vi "expressions.vi"() -> ()   [LabVIEW 2017]
uses:
  <vilib>/express/express arith-compare/Formula/XNode/ExpressFormulaBlockNode.xnode
panel:
  out "X1 2":dbl
  out "Result":dbl
  out "X1+2":dbl
  in  "X1":dbl
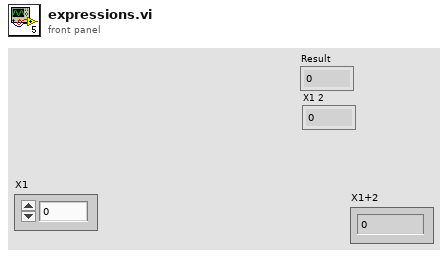
[diagram p1: front panel]
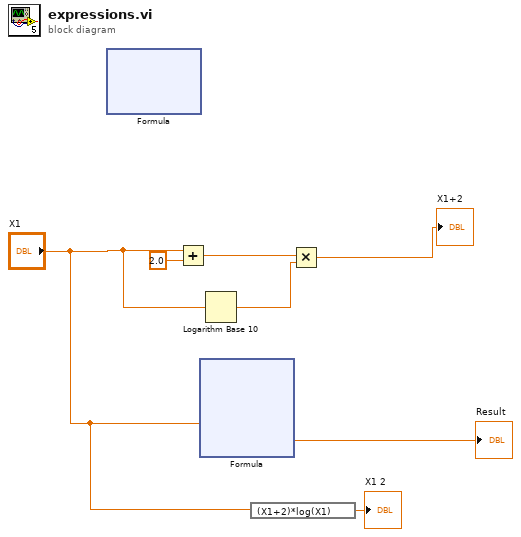
[diagram p0: block diagram]
diagram:
  n1 = xnode "Formula"() -> ()  [unwired: 2 in, 2 out]
  n2 = Add(x="X1", y=2.0) -> (x+y=w6:dbl)
  n3 = xnode "Formula"("X1"="X1") -> ("Result"=→"Result":dbl)  [unwired: 1 in, 1 out]
  n4 = Logarithm Base 10(1:"X1") -> (0:w5:dbl)
  n5 = expression code="(X1+2)*log(X1)"("X1") -> (→"X1 2":dbl)
  n6 = Multiply(x=w6, y=w5) -> (x*y=→"X1+2":dbl)
